vi "Clusters.vi"() -> ()   [LabVIEW 2020]
panel:
  out "output cluster 2":T1
  in  "Salidas Digitales":bool[](array[boolean])
  in  "Selector":u16(knob) scale=0.0..10.0
  in  "Trama JSON":string
  in  "Termocupla":dbl(slide) scale=0.0..100.0
  in  "Sendat":string
  out "output cluster":T2
  in  "Slide":dbl(slide) scale=0.0..100.0
  out "String":string
  out "Tank":dbl(slide) scale=0.0..100.0
  out "Meter":dbl(knob) scale=0.0..10.0
  out "Boolean":bool
  in  "Pesadpra de Pescado":T2 {"Variador de Velocidad" scale=0.0..10.0}
  # "Clusters"
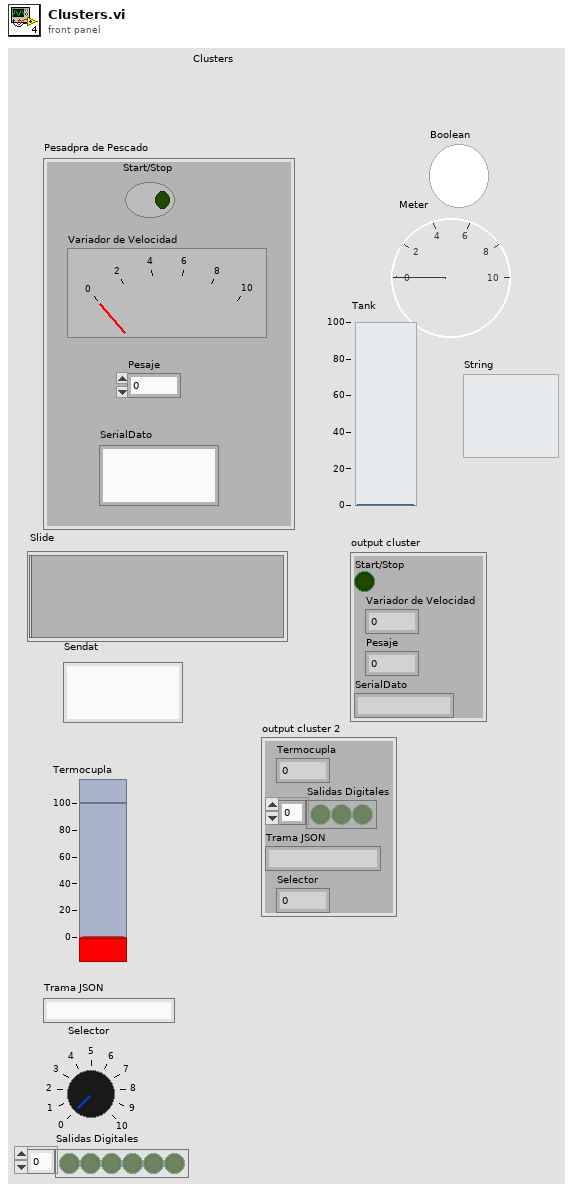
[diagram p1: front panel]
types:
  T1 = cluster{"Termocupla":dbl, "Salidas Digitales":bool[], "Trama JSON":string, "Selector":u16}
  T2 = cluster{"Start/Stop":bool, "Variador de Velocidad":dbl, "Pesaje":dbl, "SerialDato":string}
  T3 = cluster{"Data_Microcontrolador":cluster{"ADC":dbl[], "OTA":bool, "RS485_INIT":string}, "Data_PLC":cluster{"DIRECCION_IP":string, "Variadores":dbl[], "HighSpeed":i32[]}, "Trama_IOT":cluster{"Dominio":string, "PUERTO TCP":i32, "PUERTO MQTT":i32, "TOPICO":string, "TOKEN":string}, "Alarmas":cluster{"WARNING":bool[]}}
  T4 = cluster{"ADC":dbl[], "OTA":bool, "RS485_INIT":string}
  T5 = cluster{"DIRECCION_IP":string, "Variadores":dbl[], "HighSpeed":i32[]}
  T6 = cluster{"Dominio":string, "PUERTO TCP":i32, "PUERTO MQTT":i32, "TOPICO":string, "TOKEN":string}
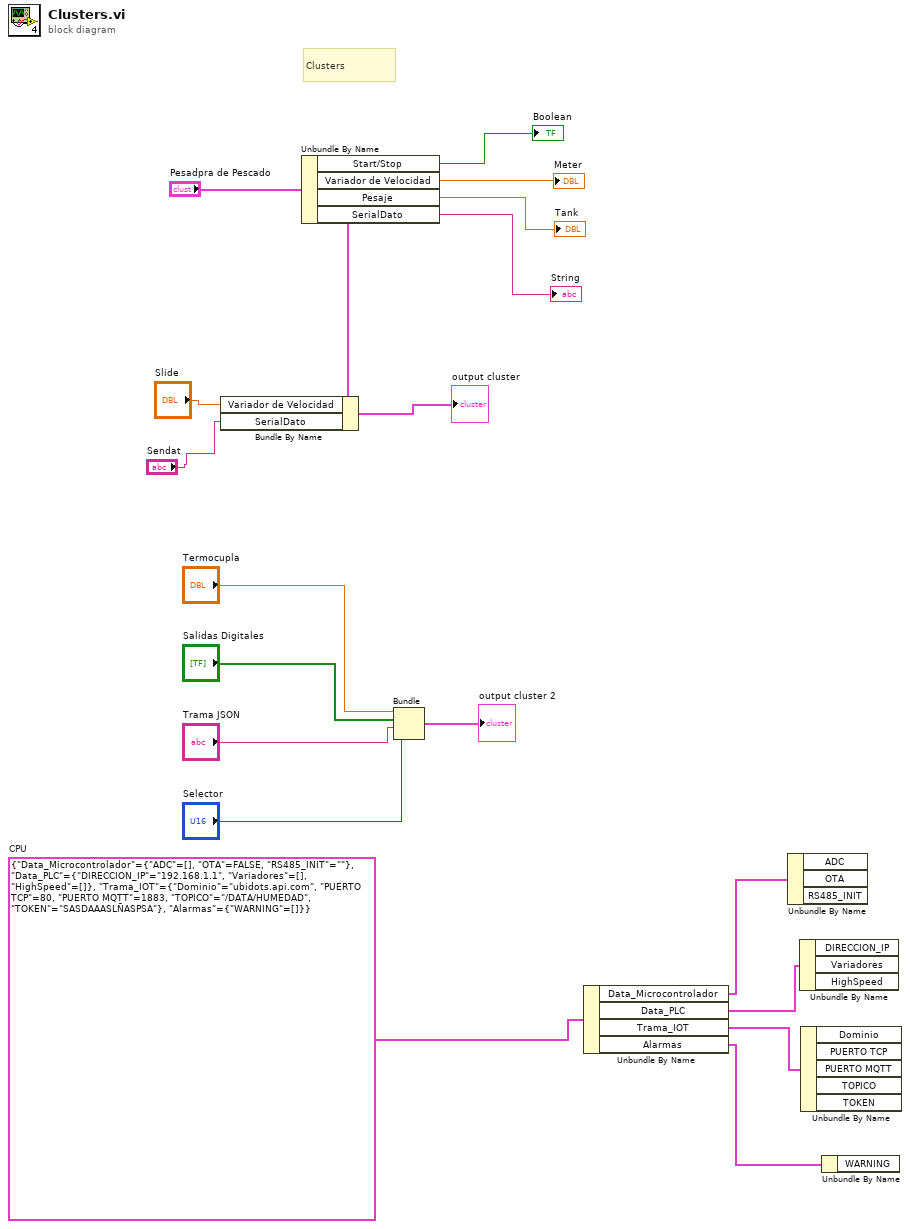
[diagram p0: block diagram]
diagram:
  w5 = T3 {"Data_Microcontrolador"={"ADC"=[], "OTA"=FALSE, "RS485_INIT"=""}, "Data_PLC"={"DIRECCION_IP"="192.168.1.1", "Variadores"=[], "HighSpeed"=[]}, "Trama_IOT"={"Dominio"="ubidots.api.com", "PUERTO TCP"=80, "PUERTO MQTT"=1883, "TOPICO"="/DATA/HUMEDAD", "TOKEN"="SASDAAASLÑASPSA"}, "Alarmas"={"WARNING"=[]}}  # CPU
  # "Clusters"
  n1 = Bundle By Name(cluster="Pesadpra de Pescado", "Variador de Velocidad"="Slide", "SerialDato"="Sendat") -> (→"output cluster":T2)
  n2 = Unbundle By Name("Pesadpra de Pescado") -> ("Start/Stop"=→"Boolean":bool, "Variador de Velocidad"=→"Meter":dbl, "Pesaje"=→"Tank":dbl, "SerialDato"=→"String":string)
  n3 = Bundle("Termocupla"="Termocupla", "Salidas Digitales"="Salidas Digitales", "Trama JSON"="Trama JSON", "Selector"="Selector") -> (→"output cluster 2":T1)  [unwired: 1 in]
  n4 = Unbundle By Name(w5) -> ("Data_Microcontrolador"=w4:T4, "Data_PLC"=w3:T5, "Trama_IOT"=w2:T6, "Alarmas"=w1:cluster{"WARNING":bool[]})
  n5 = Unbundle By Name(w4) -> ()  [unwired: 3 out]
  n6 = Unbundle By Name(w3) -> ()  [unwired: 3 out]
  n7 = Unbundle By Name(w2) -> ()  [unwired: 5 out]
  n8 = Unbundle By Name(w1) -> ()  [unwired: 1 out]
